vi "NI6343.vi"() -> ()   [LabVIEW 2014]
doc: "This program is designed for continuously acquire (Analog Input) buffered voltage measurements using a DAQmx device(NI USB 6343)."
uses:
  <vilib>/Utility/error.llb/DialogType.ctl
  <vilib>/DAQmx/create/channels.llb/DAQmx Create Channel (AI-Voltage-Basic).vi
  <vilib>/DAQmx/configure/timing.llb/DAQmx Timing (Sample Clock).vi
  <vilib>/DAQmx/read.llb/DAQmx Read (Analog 1D Wfm NChan NSamp).vi
  <resource>/objmgr/daqmx.rc
panel:
  out "Actual Sample Rate":dbl=1000.0 caption="Измеренная частота дискретизации, Гц" format="%0.2f"
  in  "REC":bool caption="Сохранить"
  in  "File Path":path=path "D:/1.tdms" caption="Путь к файлу данных"
  out "Index":i32 caption="Реализация"
  in  "Stop":bool
  out "Waveform Graph":waveform(dbl)[](graph)
  in  "Sample Rate":dbl=1000.0 caption="Частота дискретизации, Гц"
  in  "Connection Terminal":i32(ring)=-1 caption="Конфигурация подключения" items=["default"=-1, "RSE"=10083, "NRSE"=10078, "Differential"=10106, "Pseudodifferential"=12529]
  in  "Max U, В":dbl=10.0
  in  "Min U, В":dbl=-10.0
  in  "Physical channels":tag="Dev1/ai0" caption="Физические каналы"
  # "Подключение"
  # "Измеренные данные"
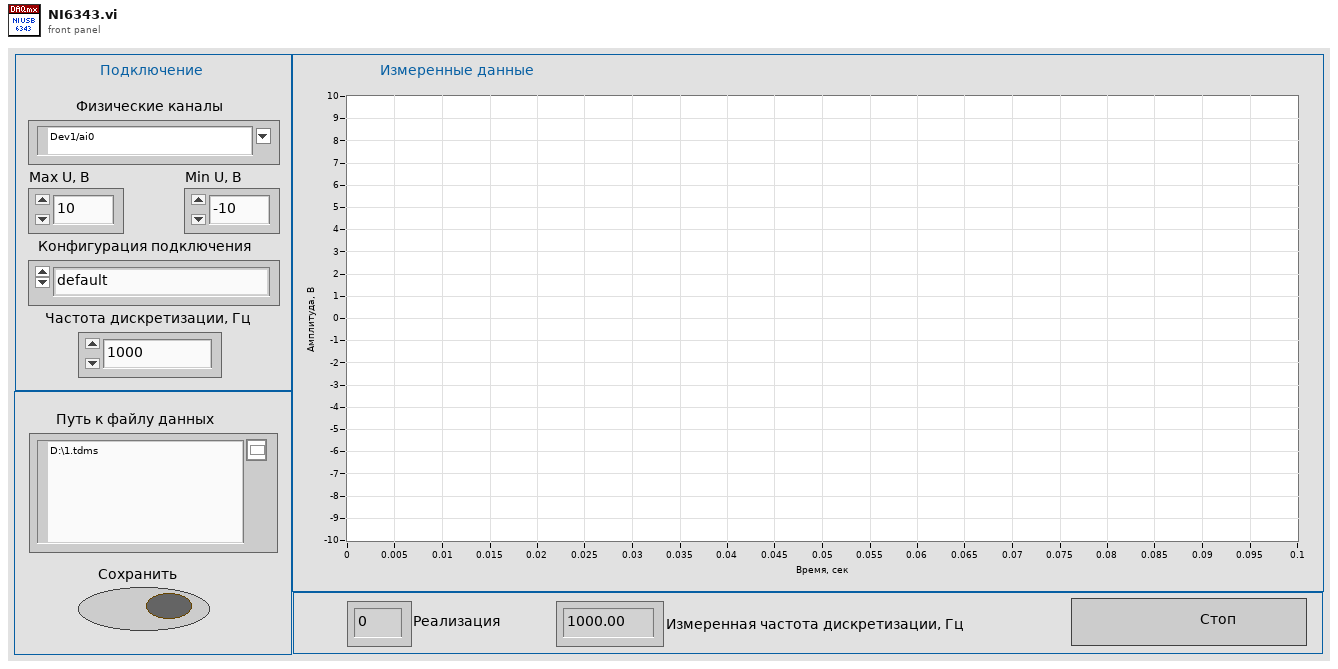
[diagram p1: front panel]
types:
  T1 = enum16{"open", "open or create", "create or replace", "create", "open (read-only)"}
  T2 = typedef "DialogType.ctl" = u16
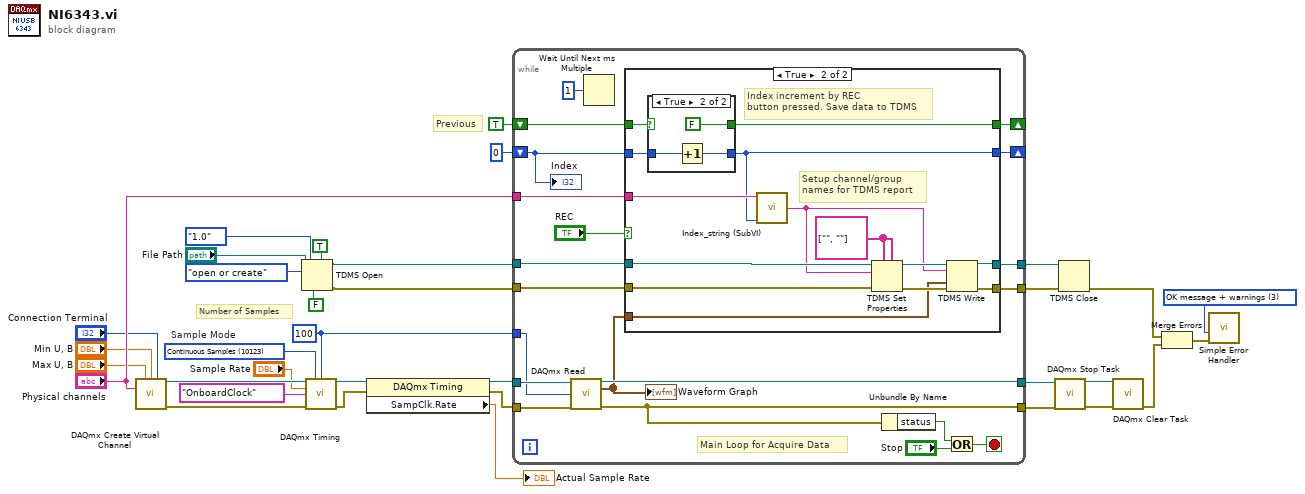
[diagram p0: block diagram]
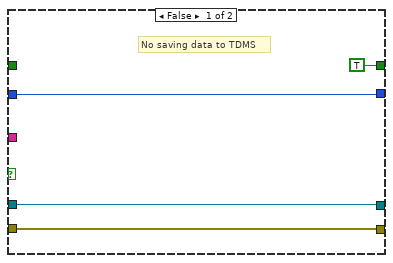
[diagram p2: hidden frame]
diagram:
  w28 = 100 ("samples per channel")
  w13 = 10123 items=["Finite Samples"=10178, "Continuous Samples"=10123, "Hardware Timed Single Point"=12522]  # Sample Mode
  w17 = T2 3 items=["no dialog", "OK message", "continue or stop message", "OK message + warnings", "continue/stop + warnings"] ("type of dialog (OK msg:1)")
  # "Number of Samples"
  # "Previous"
  n1 = call-poly <vilib>:"DAQmx Create Virtual Channel.vi"("maximum value"="Max U, В", "minimum value"="Min U, В", "input terminal configuration"="Connection Terminal", "physical channels"="Physical channels") -> ("task out"=w11:refnum<k21>, "error out"=w12:errorcluster)  [unwired: 10 in]
  n2 = TDMS Open(5:TRUE ("create index file? (T)"), 6:FALSE ("disable buffering? (T)"), 7:enum16{"1.0", "2.0"}."1.0" ("file format version (2.0)"), 10:T1."open or create" ("operation (0:open)"), 11:"File Path") -> (0:w20:errorcluster, 3:w21:refnum<k34>)  [unwired: 2 in]
  n3 = call-poly <vilib>:"DAQmx Timing.vi"("task/channels in"=w11, "sample mode"=w13, "samples per channel"=w28, "rate"="Sample Rate", "source"=tag "OnboardClock", "error in"=w12) -> ("task out"=w34:refnum<k21>, "error out"=w33:errorcluster)  [unwired: 8 in]
  n4 = property class="DAQmx Timing"(reference=w34, error in=w33) -> (reference out=w29:refnum<k21>, error out=w30:errorcluster, "SampClk.Rate"=→"Actual Sample Rate":dbl)
  n5 = while {
    tunnel: w29 -> [w48]
    tunnel: w30 -> [w54]
    tunnel: [w53] -> w32
    tunnel: [w51] -> w31
    tunnel: w28 -> [w37]
    tunnel: "Physical channels" -> [w47]
    tunnel: [w46] -> w27
    tunnel: [w45] -> w26
    tunnel: w20 -> [w44]
    tunnel: w21 -> [w43]
    shift-right: [w39] -> _
    shift-left: 0 ("samples per channel") -> [w38]
    shift-right: [w40] -> _
    shift-left: TRUE ("create index file? (T)") -> [w41]
    stop <- w49 stop-if-true
    # "Main Loop for Acquire Data"
    n6 = call-poly <vilib>:"DAQmx Read.vi"("task/channels in"=w48, "number of samples per channel"=w37, "error in"=w54) -> ("task out"=w53:refnum<k21>, "data"=w36:waveform(dbl)[], "error out"=w51:errorcluster)  [unwired: 10 in]
    "Waveform Graph" <- w36
    n7 = Wait Until Next ms Multiple(millisecond multiple=u32 1) -> ()  [unwired: 1 out]
    n8 = case shown="True" "REC" {
      tunnel: w47 -> [_ w71]
      tunnel: [w55 w68] -> w46
      tunnel: [w56 w67] -> w45
      tunnel: w44 -> [w56 w66]
      tunnel: w43 -> [w55 w65]
      tunnel: w41 -> [_ w64]
      tunnel: w38 -> [w58 w63]
      tunnel: [TRUE ("create index file? (T)") w62] -> w40
      tunnel: [w58 w61] -> w39
      tunnel: w36 -> [_ w59]
      frame False {
        # "No saving data to TDMS"
      }
      frame True {
        w72 = string[] ["", ""] ("property names")
        # "Index increment by REC\nbutton pressed. Save data to TDMS"
        # "Setup channel/group\nnames for TDMS report"
        n9 = case shown="True" w64 {
          selector: w64 -> [w74 _]
          tunnel: w63 -> [w73 w77]
          tunnel: [w74 FALSE] -> w62
          tunnel: [w73 w75] -> w61
          frame False {
          }
          frame True {
            n10 = Increment(x=w77) -> (x+1=w75:i32)
          }
        }
        n11 = call "Index_string (SubVI).vi"("Index(0..X)"=w61, "Physical Channel"=w71) -> ("Result"=w60:string)  [unwired: 2 in]
        n12 = TDMS Set Properties(5:w72, 7:w72, 8:w66, 10:w60, 11:w65) -> (0:w70:errorcluster, 3:w69:refnum<k34>)  [unwired: 1 in, 2 out]
        n13 = TDMS Write(0:w69, 5:w60, 9:w59, 11:w70) -> (4:w68:refnum<k34>, 15:w67:errorcluster)  [unwired: 2 in, 2 out]
      }
    }
    n14 = Unbundle By Name(w51) -> ("status"=w50:bool)
    n15 = Or(x=w50, y="Stop") -> (x .or. y?=w49:bool)
    "Index" <- w38
  }
  n16 = call <vilib>:"DAQmx Stop Task.vi"("task/channels in"=w32, "error in"=w31) -> ("task out"=w18:refnum<k21>, "error out"=w19:errorcluster)  [unwired: 12 in]
  n17 = TDMS Close(8:w26, 11:w27) -> (0:w14:errorcluster)  [unwired: 1 out]
  n18 = call <vilib>:"DAQmx Clear Task.vi"("task in"=w18, "error in"=w19) -> ("error out"=w15:errorcluster)  [unwired: 13 in]
  n19 = Merge Errors(w14, w15) -> (w16:errorcluster)
  n20 = call <vilib>:"Simple Error Handler.vi"("type of dialog (OK msg:1)"=w17, "error in (no error)"=w16) -> ()  [unwired: 3 in, 5 out]
